vi "test_F9P_fgv-ver.vi"() -> ()   [LabVIEW 2019] (continued)
  (unwired) cluster{"X":dbl, "Y":dbl}[] [{"X"=383412.13183575624, "Y"=283542.1157386018}, {"X"=383412.14072749903, "Y"=283542.12701954495}, {"X"=383412.14072749903, "Y"=283542.12701954495}, {"X"=383412.14072749903, "Y"=283542.12701954495}, {"X"=383412.1496192395, "Y"=283542.1383004872}, {"X"=383412.1496192395, "Y"=283542.1383004872}, {"X"=383412.1496192395, "Y"=283542.1383004872}, {"X"=383412.1496192395, "Y"=283542.1383004872}, {"X"=383412.1496192395, "Y"=283542.1383004872}, {"X"=383412.1496192395, "Y"=283542.1383004872}, {"X"=383412.1589596947, "Y"=283542.1273881729}, {"X"=383412.1589596947, "Y"=283542.1273881729}, {"X"=383412.1589596947, "Y"=283542.1273881729}, {"X"=383412.1680757925, "Y"=283542.12757248693}, {"X"=383412.1683001499, "Y"=283542.11647585774}, {"X"=383412.1774162478, "Y"=283542.11666017177}, {"X"=383412.1774162478, "Y"=283542.11666017177}, {"X"=383412.1774162478, "Y"=283542.11666017177}, {"X"=383412.18675670295, "Y"=283542.10574785754}, {"X"=383412.18675670295, "Y"=283542.10574785754}, {"X"=383412.1958728009, "Y"=283542.1059321715}, {"X"=383412.1960971583, "Y"=283542.0948355424}, {"X"=383412.20521325845, "Y"=283542.09501985647}, {"X"=383412.20521325845, "Y"=283542.09501985647}, {"X"=383412.214329354, "Y"=283542.09520417044}, {"X"=383412.214329354, "Y"=283542.09520417044}, {"X"=383412.2234454518, "Y"=283542.0953884845}, {"X"=383412.2234454518, "Y"=283542.0953884845}, {"X"=383412.2234454518, "Y"=283542.0953884845}, {"X"=383412.214329354, "Y"=283542.09520417044}, {"X"=383412.214329354, "Y"=283542.09520417044}, {"X"=383412.214329354, "Y"=283542.09520417044}, {"X"=383412.2145537114, "Y"=283542.08410754264}, {"X"=383412.20543761586, "Y"=283542.08392322867}, {"X"=383412.2056619733, "Y"=283542.0728265995}, {"X"=383412.19654587307, "Y"=283542.07264228543}, {"X"=383412.19677023054, "Y"=283542.0615456572}, {"X"=383412.0980636525, "Y"=283541.9818418036}, {"X"=383411.97245749284, "Y"=283541.87939175277}, {"X"=383411.8288434909, "Y"=283541.76547644875}, {"X"=383411.64966251695, "Y"=283541.6064373785}, {"X"=383411.4077906293, "Y"=283541.390624976}, {"X"=383411.0658659977, "Y"=283541.16168851225}, {"X"=383410.6785852051, "Y"=283540.920733869}, {"X"=383410.30953659787, "Y"=283540.6801478684}, {"X"=383409.922704477, "Y"=283540.41700000333}, {"X"=383409.49985664326, "Y"=283540.1309216538}, {"X"=383409.04943613, "Y"=283539.85538702144}, {"X"=383408.5990155877, "Y"=283539.5798524129}, {"X"=383408.15771112393, "Y"=283539.30450213735}, {"X"=383407.7252983808, "Y"=283539.0404328218}, {"X"=383407.30200171185, "Y"=283538.7765478377}, {"X"=383406.8962641739, "Y"=283538.54632137535}, {"X"=383406.4998670677, "Y"=283538.3051826139}, {"X"=383406.10369428596, "Y"=283538.05294724106}, {"X"=383405.6895136327, "Y"=283537.7892466443}, {"X"=383405.28444905346, "Y"=283537.52573037276}, {"X"=383404.870044003, "Y"=283537.2731264438}, {"X"=383404.4554145847, "Y"=283537.0316191623}, {"X"=383404.04100949224, "Y"=283536.77901527355}, {"X"=383403.6266043726, "Y"=283536.52641140413}, {"X"=383403.18529961235, "Y"=283536.2510613829}, {"X"=383402.7346543793, "Y"=283535.9866237099}, {"X"=383402.29312522465, "Y"=283535.72237036366}, {"X"=383401.85182039154, "Y"=283535.44702041155}, {"X"=383401.43763949943, "Y"=283535.18332001864}, {"X"=383401.0603716887, "Y"=283534.89816360164}, {"X"=383400.74758961983, "Y"=283534.58100742893}, {"X"=383400.4815097676, "Y"=283534.2092896391}, {"X"=383400.280140006, "Y"=283533.79447545746}, {"X"=383400.14348033105, "Y"=283533.33656487794}, {"X"=383400.07197944535, "Y"=283532.81336464395}, {"X"=383400.0834208813, "Y"=283532.24743661174}, {"X"=383400.18602339644, "Y"=283531.68335159513}, {"X"=383400.41512973054, "Y"=283531.17732994177}, {"X"=383400.72426198516, "Y"=283530.7728366644}, {"X"=383401.0771800759, "Y"=283530.4580379334}, {"X"=383401.45587610855, "Y"=283530.2214685208}, {"X"=383401.88792276254, "Y"=283530.0525847101}, {"X"=383402.30928290833, "Y"=283529.9611930121}, {"X"=383402.7477535631, "Y"=283529.9256530838}, {"X"=383403.16642158024, "Y"=283529.9674209622}, {"X"=383403.52904686355, "Y"=283530.07466280117}, {"X"=383403.90878262615, "Y"=283530.2377564051}, {"X"=383404.31496931607, "Y"=283530.44578945445}, {"X"=383404.7382664643, "Y"=283530.7096742769}, {"X"=383405.1704553586, "Y"=283530.9848400567}, {"X"=383405.5937524603, "Y"=283531.2487249207}, {"X"=383405.99926602206, "Y"=283531.4900479345}, {"X"=383406.3954391052, "Y"=283531.7422832877}, {"X"=383406.81828743755, "Y"=283532.02836147026}, {"X"=383407.25002750533, "Y"=283532.3257206095}, {"X"=383407.6726514358, "Y"=283532.6228954618}, {"X"=383408.0954996884, "Y"=283532.9089737058}, {"X"=383408.5456962394, "Y"=283533.19560490194}, {"X"=383408.98655230104, "Y"=283533.4931484379}, {"X"=383409.40962482896, "Y"=283533.7681301187}, {"X"=383409.81446512, "Y"=283534.0427432001}, {"X"=383410.2101892815, "Y"=283534.3171719865}, {"X"=383410.6150295247, "Y"=283534.5917851032}, {"X"=383411.02898584673, "Y"=283534.86658255244}, {"X"=383411.4431665024, "Y"=283535.1302833934}, {"X"=383411.8575714911, "Y"=283535.3828876251}, {"X"=383412.28975995193, "Y"=283535.65805376216}, {"X"=383412.7401805953, "Y"=283535.9335885495}, {"X"=383413.1632529006, "Y"=283536.20857041556}, {"X"=383413.5772090795, "Y"=283536.48336798773}, {"X"=383414.00028133026, "Y"=283536.75834989623}, {"X"=383414.47737710393, "Y"=283537.0677276065}, {"X"=383414.95424848073, "Y"=283537.38820197195}, {"X"=383415.36775582953, "Y"=283537.6851928882}, {"X"=383415.72634217737, "Y"=283537.9921745477}, {"X"=383416.0202183364, "Y"=283538.3422525123}, {"X"=383416.2673921541, "Y"=283538.74689204094}, {"X"=383416.4496314275, "Y"=283539.2057244933}, {"X"=383416.54870396585, "Y"=283539.7183812282}, {"X"=383416.5472750222, "Y"=283540.24010709027}, {"X"=383416.48270647053, "Y"=283540.7272528411}, {"X"=383416.3369904831, "Y"=283541.1683532132}, {"X"=383416.1096783414, "Y"=283541.5856014671}, {"X"=383415.8103348771, "Y"=283541.95698867145}, {"X"=383415.43006836623, "Y"=283542.2712338854}, {"X"=383414.9873353622, "Y"=283542.51760912524}, {"X"=383414.50993287616, "Y"=283542.67447409057}, {"X"=383414.0436657404, "Y"=283542.73165373795}, {"X"=383413.5880852258, "Y"=283542.7113413258}, {"X"=383413.1160673846, "Y"=283542.60188727773}, {"X"=383412.6638522345, "Y"=283542.41512548324}, {"X"=383412.2316641198, "Y"=283542.1399593133}, {"X"=383412.1058336066, "Y"=283542.04860588827}, {"X"=383412.09671750874, "Y"=283542.04842157435}, {"X"=383412.1058336066, "Y"=283542.04860588827}, {"X"=383412.1149497068, "Y"=283542.04879020224}, {"X"=383412.12406580243, "Y"=283542.04897451616}, {"X"=383412.13295754296, "Y"=283542.0602554593}, {"X"=383412.13295754296, "Y"=283542.0602554593}, {"X"=383412.14207364316, "Y"=283542.06043977325}, {"X"=383412.1511897411, "Y"=283542.06062408723}, {"X"=383412.160305839, "Y"=283542.0608084012}]  # wpt_polypusan_20200714-3
  (unwired) cluster{"X":dbl, "Y":dbl}[] [{"X"=383411.932320843, "Y"=283542.5113466384}, {"X"=383411.94143694045, "Y"=283542.5115309522}, {"X"=383411.9503286807, "Y"=283542.5228118937}, {"X"=383411.95944477816, "Y"=283542.5229962075}, {"X"=383411.96856087557, "Y"=283542.5231805213}, {"X"=383411.9683365184, "Y"=283542.53427715093}, {"X"=383411.9774526181, "Y"=283542.5344614648}, {"X"=383411.9865687132, "Y"=283542.53464577853}, {"X"=383411.9956848153, "Y"=283542.5348300925}, {"X"=383411.8696299463, "Y"=283542.4545732997}, {"X"=383411.6993407283, "Y"=283542.3068151703}, {"X"=383411.54683498706, "Y"=283542.18161892693}, {"X"=383411.37654576113, "Y"=283542.0338608031}, {"X"=383411.1517842929, "Y"=283541.87390017736}, {"X"=383410.8998988804, "Y"=283541.7022899903}, {"X"=383410.62978125946, "Y"=283541.5303111862}, {"X"=383410.3509962426, "Y"=283541.33595482114}, {"X"=383410.072211214, "Y"=283541.1415984661}, {"X"=383409.7754183256, "Y"=283540.9357768668}, {"X"=383409.4697336811, "Y"=283540.71867434034}, {"X"=383409.146265533, "Y"=283540.47900994436}, {"X"=383408.83146475896, "Y"=283540.26172312885}, {"X"=383408.5526796635, "Y"=283540.0673668221}, {"X"=383408.28256195365, "Y"=283539.8953880912}, {"X"=383408.0122198793, "Y"=283539.7345059978}, {"X"=383407.7872339495, "Y"=283539.5856420879}, {"X"=383407.6249389544, "Y"=283539.4935514922}, {"X"=383407.4177365061, "Y"=283539.36724946724}, {"X"=383407.18341010157, "Y"=283539.2292978924}, {"X"=383406.9399675942, "Y"=283539.0911620164}, {"X"=383406.6513932718, "Y"=283538.92991135013}, {"X"=383406.33591933665, "Y"=283538.74591451185}, {"X"=383405.98465403315, "Y"=283538.5278905661}, {"X"=383405.6333887108, "Y"=283538.3098666383}, {"X"=383405.2641155198, "Y"=283538.080377482}, {"X"=383404.8590509454, "Y"=283537.8168612309}, {"X"=383404.4450945958, "Y"=283537.54206406383}, {"X"=383404.04025432153, "Y"=283537.2674512232}, {"X"=383403.6443057818, "Y"=283537.00411933445}, {"X"=383403.2485815608, "Y"=283536.7296908353}, {"X"=383402.85263297544, "Y"=283536.4663589834}, {"X"=383402.4389008485, "Y"=283536.18046528485}, {"X"=383402.025168696, "Y"=283535.89457160764}, {"X"=383401.6474522479, "Y"=283535.6316084193}, {"X"=383401.2877436384, "Y"=283535.38011048}, {"X"=383400.94694025436, "Y"=283535.0956912774}, {"X"=383400.62571511255, "Y"=283534.74506092304}, {"X"=383400.3509678404, "Y"=283534.35096557817}, {"X"=383400.140930653, "Y"=283533.9137738416}, {"X"=383399.99582789536, "Y"=283533.42238907877}, {"X"=383399.9518996638, "Y"=283532.8886451223}, {"X"=383399.9995811818, "Y"=283532.33455092355}, {"X"=383400.1475398879, "Y"=283531.782484042}, {"X"=383400.4042188871, "Y"=283531.26591866364}, {"X"=383400.7318076984, "Y"=283530.8506973626}, {"X"=383401.120965875, "Y"=283530.54773247044}, {"X"=383401.56325033365, "Y"=283530.32354980666}, {"X"=383402.03998015146, "Y"=283530.1999740305}, {"X"=383402.5151395754, "Y"=283530.15407467587}, {"X"=383402.9796124794, "Y"=283530.1856674368}, {"X"=383403.4247314314, "Y"=283530.2723747546}, {"X"=383403.85004773084, "Y"=283530.4363898795}, {"X"=383404.2922501598, "Y"=283530.6673534074}, {"X"=383404.74311997613, "Y"=283530.92069452035}, {"X"=383405.16664144257, "Y"=283531.17348273523}, {"X"=383405.61751120875, "Y"=283531.42682389263}, {"X"=383406.08594012377, "Y"=283531.7138235732}, {"X"=383406.5452528999, "Y"=283532.00063897157}, {"X"=383407.04013267846, "Y"=283532.33257814153}, {"X"=383407.5619120408, "Y"=283532.6872635217}, {"X"=383408.092583116, "Y"=283533.0532298735}, {"X"=383408.5968032415, "Y"=283533.37425681524}, {"X"=383409.08279111754, "Y"=283533.69491516484}, {"X"=383409.5692276718, "Y"=283533.9933802838}, {"X"=383410.10057165544, "Y"=283534.3260568743}, {"X"=383410.6854904599, "Y"=283534.7153225135}, {"X"=383411.26106875925, "Y"=283535.11550050834}, {"X"=383411.8279796103, "Y"=283535.493300969}, {"X"=383412.34998296807, "Y"=283535.83689001354}, {"X"=383412.82707883895, "Y"=283536.14626763324}, {"X"=383413.3495308398, "Y"=283536.4676634827}, {"X"=383413.89021501347, "Y"=283536.7894279925}, {"X"=383414.3762025273, "Y"=283537.11008664395}, {"X"=383414.844182165, "Y"=283537.4192800597}, {"X"=383415.32082914957, "Y"=283537.7508510744}, {"X"=383415.7781220907, "Y"=283538.1375366228}, {"X"=383416.1426834359, "Y"=283538.6000554199}, {"X"=383416.40562146157, "Y"=283539.12712650327}, {"X"=383416.53981222806, "Y"=283539.7071002825}, {"X"=383416.57305278804, "Y"=283540.31833644706}, {"X"=383416.451319649, "Y"=283540.92643920117}, {"X"=383416.2213151491, "Y"=283541.47684699734}, {"X"=383415.8748206522, "Y"=283541.92498900933}, {"X"=383415.43006836623, "Y"=283542.2712338854}, {"X"=383414.93241441366, "Y"=283542.5275998535}, {"X"=383414.4092070801, "Y"=283542.694639868}, {"X"=383413.8978081814, "Y"=283542.7287046846}, {"X"=383413.33350757346, "Y"=283542.6728906116}, {"X"=383412.79879883706, "Y"=283542.50666323025}, {"X"=383412.3112410692, "Y"=283542.2636810541}, {"X"=383412.1309383268, "Y"=283542.1601251152}, {"X"=383412.1222709437, "Y"=283542.13774754526}, {"X"=383412.1222709437, "Y"=283542.13774754526}, {"X"=383412.1316113989, "Y"=283542.12683523097}, {"X"=383412.1316113989, "Y"=283542.12683523097}, {"X"=383412.1316113989, "Y"=283542.12683523097}, {"X"=383412.1316113989, "Y"=283542.12683523097}, {"X"=383412.1316113989, "Y"=283542.12683523097}, {"X"=383412.14072749903, "Y"=283542.12701954495}, {"X"=383412.14984359685, "Y"=283542.1272038589}]  # poly pusan 20200714-2
  (unwired) cluster{"X":dbl, "Y":dbl}[] [{"X"=383409.9178374654, "Y"=283536.59810102}, {"X"=383409.927177923, "Y"=283536.58718870144}, {"X"=383409.93651838053, "Y"=283536.57627638616}, {"X"=383409.9549749438, "Y"=283536.5655483811}, {"X"=383409.96431539906, "Y"=283536.55463606486}, {"X"=383409.973655859, "Y"=283536.5437237469}, {"X"=383409.98277195997, "Y"=283536.54390805843}, {"X"=383409.9469806094, "Y"=283536.50988092675}, {"X"=383409.93831321446, "Y"=283536.4875033598}, {"X"=383409.9385375687, "Y"=283536.4764067302}, {"X"=383409.9385375687, "Y"=283536.4764067302}, {"X"=383409.93876192294, "Y"=283536.4653101011}, {"X"=383409.8578387605, "Y"=283536.40816815686}, {"X"=383409.7769156017, "Y"=283536.35102621204}, {"X"=383409.7589077463, "Y"=283536.3395609602}, {"X"=383409.73200814123, "Y"=283536.3168147713}, {"X"=383409.5792779161, "Y"=283536.20271519583}, {"X"=383409.27336874546, "Y"=283535.99670931126}, {"X"=383408.841180219, "Y"=283535.72154332086}, {"X"=383408.3816433538, "Y"=283535.4458244228}, {"X"=383408.05727756815, "Y"=283535.25054659066}, {"X"=383407.9223308085, "Y"=283535.15900892194}, {"X"=383407.94056302006, "Y"=283535.15937754087}, {"X"=383408.09396634065, "Y"=283535.2401872}, {"X"=383408.3194010837, "Y"=283535.36685785564}, {"X"=383408.61776466237, "Y"=283535.4950029968}, {"X"=383409.05421591504, "Y"=283535.55933303706}, {"X"=383409.60140653874, "Y"=283535.55929506075}, {"X"=383410.21285860625, "Y"=283535.5383540437}, {"X"=383410.69646085746, "Y"=283535.52592932346}, {"X"=383410.96971964114, "Y"=283535.5425553223}, {"X"=383411.1155773138, "Y"=283535.5455043238}, {"X"=383411.3519229675, "Y"=283535.5835863414}, {"X"=383411.5695876939, "Y"=283535.64349299634}, {"X"=383411.6963157314, "Y"=283535.69045989437}, {"X"=383411.94954744837, "Y"=283535.7954903261}, {"X"=383412.0940589766, "Y"=283535.86501911347}, {"X"=383412.17520648835, "Y"=283535.9110644512}, {"X"=383412.2472378928, "Y"=283535.95692547486}, {"X"=383412.2743618502, "Y"=283535.9685750442}, {"X"=383412.2743618502, "Y"=283535.9685750442}, {"X"=383412.2741374931, "Y"=283535.9796716734}, {"X"=383412.2741374931, "Y"=283535.9796716734}, {"X"=383412.2741374931, "Y"=283535.9796716734}, {"X"=383412.2741374931, "Y"=283535.9796716734}, {"X"=383412.2741374931, "Y"=283535.9796716734}, {"X"=383412.2741374931, "Y"=283535.9796716734}, {"X"=383412.2741374931, "Y"=283535.9796716734}, {"X"=383412.2741374931, "Y"=283535.9796716734}, {"X"=383412.2743618502, "Y"=283535.9685750442}, {"X"=383412.26524574624, "Y"=283535.9683907304}, {"X"=383412.2650213891, "Y"=283535.9794873595}, {"X"=383412.2650213891, "Y"=283535.9794873595}, {"X"=383412.2559052828, "Y"=283535.97930304566}, {"X"=383412.291920987, "Y"=283536.0022335576}, {"X"=383412.53581222554, "Y"=283536.11817631975}, {"X"=383412.77970346273, "Y"=283536.2341190897}, {"X"=383412.987578986, "Y"=283536.3271313491}, {"X"=383413.19545451214, "Y"=283536.42014361545}, {"X"=383413.367089974, "Y"=283536.5013219984}, {"X"=383413.49336927186, "Y"=283536.5704821794}, {"X"=383413.5293849731, "Y"=283536.59341269743}, {"X"=383413.5385010765, "Y"=283536.5935970126}, {"X"=383413.5567332834, "Y"=283536.5939656429}, {"X"=383413.56584938685, "Y"=283536.59414995805}, {"X"=383413.5749654926, "Y"=283536.59433427325}, {"X"=383413.71013653226, "Y"=283536.6747754009}, {"X"=383414.22324801044, "Y"=283537.0070836166}, {"X"=383414.9242078476, "Y"=283537.5208085642}, {"X"=383415.63002084335, "Y"=283538.2455538307}, {"X"=383416.1836939611, "Y"=283539.2780556692}, {"X"=383416.2779721501, "Y"=283540.4788876928}, {"X"=383415.9344532047, "Y"=283541.68196908606}, {"X"=383415.1402897733, "Y"=283542.62061217}, {"X"=383414.0938751328, "Y"=283542.95469220664}, {"X"=383413.47308307973, "Y"=283542.9865452564}, {"X"=383413.3452333581, "Y"=283542.9950614707}, {"X"=383413.3267768075, "Y"=283543.0057894686}, {"X"=383413.3174363517, "Y"=283543.01670178166}, {"X"=383413.38102467154, "Y"=283543.0290886174}, {"X"=383413.9084121501, "Y"=283543.1063586886}, {"X"=383414.70860945265, "Y"=283543.2224481709}, {"X"=383414.95384662825, "Y"=283543.2718112374}, {"X"=383414.95362226735, "Y"=283543.2829078666}, {"X"=383414.9533979065, "Y"=283543.2940044949}, {"X"=383414.9531735456, "Y"=283543.3051011227}, {"X"=383414.9169335171, "Y"=283543.29326722753}, {"X"=383414.6076593038, "Y"=283543.25371057465}, {"X"=383413.9711030325, "Y"=283543.1631320421}, {"X"=383413.3634655521, "Y"=283542.9954301012}, {"X"=383412.93972051237, "Y"=283542.7537380956}, {"X"=383412.5989177596, "Y"=283542.4693184259}, {"X"=383412.09537136485, "Y"=283542.11500134604}, {"X"=383411.53690398356, "Y"=283541.77067504416}, {"X"=383411.0869323256, "Y"=283541.47294704843}, {"X"=383410.7814720845, "Y"=283541.2447478443}, {"X"=383410.583610174, "Y"=283541.1075334294}, {"X"=383410.466222666, "Y"=283541.04965422716}, {"X"=383410.4297582683, "Y"=283541.04891697824}, {"X"=383410.41130171315, "Y"=283541.059644982}, {"X"=383410.8434899318, "Y"=283541.33481106185}, {"X"=383411.3746090679, "Y"=283541.67858437833}, {"X"=383411.8963877096, "Y"=283542.03327004256}, {"X"=383412.49042201624, "Y"=283542.42272013833}, {"X"=383413.04044630117, "Y"=283542.7335723024}, {"X"=383413.4459591501, "Y"=283542.9748956804}, {"X"=383413.81545630284, "Y"=283543.1932885606}, {"X"=383414.26654959243, "Y"=283543.4355335569}, {"X"=383414.59158803057, "Y"=283543.59752174537}, {"X"=383414.6727354587, "Y"=283543.6435671087}, {"X"=383414.6725110981, "Y"=283543.65466373705}, {"X"=383414.663395004, "Y"=283543.6544794205}, {"X"=383414.5277753554, "Y"=283543.59623153013}, {"X"=383414.39215570525, "Y"=283543.53798364184}, {"X"=383414.1751642665, "Y"=283543.4447870245}, {"X"=383413.7863131391, "Y"=283543.2815086416}, {"X"=383413.42548336374, "Y"=283543.085493336}, {"X"=383413.1546927557, "Y"=283542.94680433837}, {"X"=383412.9650495782, "Y"=283542.854160697}, {"X"=383412.7938629567, "Y"=283542.75078906}, {"X"=383412.56865281187, "Y"=283542.6130216534}, {"X"=383412.41547401866, "Y"=283542.52111528144}, {"X"=383412.37056660216, "Y"=283542.48690382455}, {"X"=383412.36167486466, "Y"=283542.47562288266}, {"X"=383412.28120048554, "Y"=283542.39628765377}, {"X"=383412.2182852302, "Y"=283542.3506109417}, {"X"=383412.2091691326, "Y"=283542.3504266277}, {"X"=383412.2093934901, "Y"=283542.33932999894}, {"X"=383412.2093934901, "Y"=283542.33932999894}, {"X"=383412.2093934901, "Y"=283542.33932999894}, {"X"=383412.2093934901, "Y"=283542.33932999894}, {"X"=383412.2463065955, "Y"=283542.3178739988}, {"X"=383412.2554226954, "Y"=283542.31805831287}, {"X"=383412.2645387931, "Y"=283542.31824262696}, {"X"=383412.2738792506, "Y"=283542.3073303115}, {"X"=383412.1665052908, "Y"=283542.2052488859}, {"X"=383411.77922457363, "Y"=283541.9642941928}, {"X"=383411.38305209693, "Y"=283541.71205857664}, {"X"=383411.10381838854, "Y"=283541.5398954449}, {"X"=383410.8697164487, "Y"=283541.3908471426}, {"X"=383410.6447306024, "Y"=283541.2419831568}, {"X"=383410.41062864766, "Y"=283541.0929348684}, {"X"=383410.14940274344, "Y"=283540.9322370196}, {"X"=383409.9155251322, "Y"=283540.77209211467}, {"X"=383409.6903149036, "Y"=283540.6343247839}, {"X"=383409.43842942733, "Y"=283540.4627146399}, {"X"=383409.24056747806, "Y"=283540.3255002548}, {"X"=383409.17765219585, "Y"=283540.27982356516}, {"X"=383409.2585753234, "Y"=283540.3369655045}, {"X"=383409.5375847504, "Y"=283540.52022520616}, {"X"=383409.8617259532, "Y"=283540.7265997316}, {"X"=383410.20365063194, "Y"=283540.95553614816}, {"X"=383410.608939274, "Y"=283541.20795602264}, {"X"=383410.995546983, "Y"=283541.4822005473}, {"X"=383411.3283555053, "Y"=283541.7109526976}, {"X"=383411.68873666425, "Y"=283541.9291611722}, {"X"=383411.95862989506, "Y"=283542.1122366382}, {"X"=383412.12070044235, "Y"=283542.2154239456}, {"X"=383412.1567161209, "Y"=283542.2383544585}, {"X"=383412.1658322186, "Y"=283542.23853877245}, {"X"=383412.1658322186, "Y"=283542.23853877245}, {"X"=383412.1749483163, "Y"=283542.2387230865}, {"X"=383412.1749483163, "Y"=283542.2387230865}, {"X"=383412.2025209692, "Y"=283542.2281793989}, {"X"=383412.2025209692, "Y"=283542.2281793989}, {"X"=383412.2025209692, "Y"=283542.2281793989}, {"X"=383412.21163706464, "Y"=283542.22836371296}, {"X"=383412.21163706464, "Y"=283542.22836371296}, {"X"=383412.22052880493, "Y"=283542.2396446566}, {"X"=383412.22052880493, "Y"=283542.2396446566}, {"X"=383412.18496184365, "Y"=283542.1945208857}, {"X"=383412.09537136485, "Y"=283542.11500134604}, {"X"=383411.9788813051, "Y"=283542.0127356099}, {"X"=383411.8530507877, "Y"=283541.9213821895}, {"X"=383411.67274803354, "Y"=283541.8178262597}, {"X"=383411.46532133967, "Y"=283541.7026207666}, {"X"=383411.29413467535, "Y"=283541.59924916073}, {"X"=383411.1767471755, "Y"=283541.54136994836}, {"X"=383411.07759187114, "Y"=283541.48385936284}, {"X"=383410.9510882701, "Y"=283541.42579584295}, {"X"=383410.80702553515, "Y"=283541.33407381136}, {"X"=383410.6173823041, "Y"=283541.24143021955}, {"X"=383410.48198695586, "Y"=283541.1720857659}, {"X"=383410.4457469139, "Y"=283541.16025188734}, {"X"=383410.43663081515, "Y"=283541.1600675751}, {"X"=383410.3557076998, "Y"=283541.1029256232}, {"X"=383410.1934127563, "Y"=283541.0108349785}, {"X"=383410.0039938697, "Y"=283540.90709477285}, {"X"=383409.7696675421, "Y"=283540.769143129}, {"X"=383409.53511685575, "Y"=283540.6422881183}, {"X"=383409.3730462501, "Y"=283540.53910085984}, {"X"=383409.2380995876, "Y"=283540.44756316737}, {"X"=383409.04912938597, "Y"=283540.3216297263}, {"X"=383408.81480303186, "Y"=283540.1836781074}, {"X"=383408.55402578035, "Y"=283540.00078705046}, {"X"=383408.26590022095, "Y"=283539.817343072}, {"X"=383407.9686585453, "Y"=283539.63371479337}, {"X"=383407.67141686263, "Y"=283539.450086526}, {"X"=383407.3743995172, "Y"=283539.2553616379}, {"X"=383407.05025820807, "Y"=283539.0489872076}, {"X"=383406.71700078365, "Y"=283538.8424284801}, {"X"=383406.3926350932, "Y"=283538.64715070394}, {"X"=383406.04159413883, "Y"=283538.41803012847}, {"X"=383405.7174527709, "Y"=283538.2116557487}, {"X"=383405.4113192408, "Y"=283538.01674662315}, {"X"=383405.0869534989, "Y"=283537.8214688956}, {"X"=383404.7810442931, "Y"=283537.615463163}, {"X"=383404.4840268283, "Y"=283537.4207383768}, {"X"=383404.21413331095, "Y"=283537.2376631467}, {"X"=383403.9440154383, "Y"=283537.06568455126}, {"X"=383403.65588969685, "Y"=283536.8822407282}, {"X"=383403.36753959535, "Y"=283536.70989354217}, {"X"=383403.0525142093, "Y"=283536.5037035683}, {"X"=383402.692581331, "Y"=283536.26330219803}, {"X"=383402.3237566754, "Y"=283536.0116199123}, {"X"=383401.990947726, "Y"=283535.7828681109}, {"X"=383401.75729418325, "Y"=283535.61162680085}, {"X"=383401.6312391361, "Y"=283535.5313701584}, {"X"=383401.4962923195, "Y"=283535.4398325877}, {"X"=383401.2984301499, "Y"=283535.30261838617}, {"X"=383401.0827844499, "Y"=283535.1428423272}, {"X"=383400.8944870562, "Y"=283534.98361918115}, {"X"=383400.70641399856, "Y"=283534.8132994113}, {"X"=383400.5010060944, "Y"=283534.5982245295}, {"X"=383400.3060603416, "Y"=283534.3167541855}, {"X"=383400.13958460063, "Y"=283533.9803536106}, {"X"=383400.00157887576, "Y"=283533.5890228039}, {"X"=383399.91049971955, "Y"=283533.1320337348}, {"X"=383399.89302243193, "Y"=283532.64322919585}, {"X"=383399.93890921294, "Y"=283532.17790802126}, {"X"=383400.04703835654, "Y"=283531.79155335313}, {"X"=383400.18049675727, "Y"=283531.50562124373}, {"X"=383400.30304432334, "Y"=283531.3082778588}, {"X"=383400.38800574763, "Y"=283531.1656804091}, {"X"=383400.50053984235, "Y"=283531.0125392357}, {"X"=383400.68712452496, "Y"=283530.8053893417}, {"X"=383400.8917170911, "Y"=283530.60970468115}, {"X"=383401.1596737439, "Y"=283530.43750339915}, {"X"=383401.4545300481, "Y"=283530.2880482896}, {"X"=383401.78517776896, "Y"=283530.17262028495}, {"X"=383402.16984912794, "Y"=283530.09158799663}, {"X"=383402.58052275726, "Y"=283530.07768840576}, {"X"=383402.9811828962, "Y"=283530.1079910402}, {"X"=383403.37115650147, "Y"=283530.2157857858}, {"X"=383403.8138076402, "Y"=283530.42455603235}, {"X"=383404.3193741375, "Y"=283530.6790029523}, {"X"=383404.7793600638, "Y"=283530.93252837134}, {"X"=383405.14863357117, "Y"=283531.1620174932}, {"X"=383405.4187516078, "Y"=283531.3339961164}, {"X"=383405.5988302973, "Y"=283531.4486485354}, {"X"=383405.77868462657, "Y"=283531.5743975866}, {"X"=383405.95876330684, "Y"=283531.6890500145}, {"X"=383406.19264122855, "Y"=283531.8491948027}, {"X"=383406.51633412845, "Y"=283532.0777624464}, {"X"=383406.8495918177, "Y"=283532.2843211534}, {"X"=383407.1286015494, "Y"=283532.4675807652}, {"X"=383407.4076112677, "Y"=283532.650840386}, {"X"=383407.70485319116, "Y"=283532.83446863596}, {"X"=383408.00187074905, "Y"=283533.0291935228}, {"X"=383408.3353527256, "Y"=283533.2246556581}, {"X"=383408.66838598094, "Y"=283533.44231106626}, {"X"=383408.97474396054, "Y"=283533.6261236677}, {"X"=383409.27176146646, "Y"=283533.8208486002}, {"X"=383409.61368643295, "Y"=283534.04978498194}, {"X"=383410.0009675565, "Y"=283534.2907395623}, {"X"=383410.39736476535, "Y"=283534.5318784738}, {"X"=383410.76641363365, "Y"=283534.7724644647}, {"X"=383411.117454633, "Y"=283535.0015852203}, {"X"=383411.4778360758, "Y"=283535.2197936726}, {"X"=383411.8831249549, "Y"=283535.4722135931}, {"X"=383412.2695085299, "Y"=283535.75755479146}, {"X"=383412.6385573031, "Y"=283535.9981408621}, {"X"=383412.9624742541, "Y"=283536.21561212145}, {"X"=383413.2866155505, "Y"=283536.4219867639}, {"X"=383413.62876467826, "Y"=283536.6398266781}, {"X"=383413.9800298931, "Y"=283536.85785092146}, {"X"=383414.3404111968, "Y"=283537.0760594928}, {"X"=383414.6736685308, "Y"=283537.28261850367}, {"X"=383414.979801905, "Y"=283537.47752794967}, {"X"=383415.28571090545, "Y"=283537.6835340353}, {"X"=383415.5911711697, "Y"=283537.91173338844}, {"X"=383415.88616914465, "Y"=283538.20632820437}, {"X"=383416.1620374513, "Y"=283538.5449409112}, {"X"=383416.38231168006, "Y"=283538.92683423456}, {"X"=383416.54744055454, "Y"=283539.3298149099}, {"X"=383416.64808362443, "Y"=283539.764795244}, {"X"=383416.66623305104, "Y"=283540.22030997305}, {"X"=383416.6021132184, "Y"=283540.6852624638}, {"X"=383416.4381650218, "Y"=283541.1259941986}, {"X"=383416.22930943617, "Y"=283541.53251445986}, {"X"=383415.9393064278, "Y"=283541.89298934815}, {"X"=383415.58638820087, "Y"=283542.2077875092}, {"X"=383415.21680833364, "Y"=283542.4445406474}, {"X"=383414.83945855283, "Y"=283542.6145297139}, {"X"=383414.4547875691, "Y"=283542.6955614495}, {"X"=383414.0258822629, "Y"=283542.70909185003}, {"X"=383413.5434021757, "Y"=283542.6660332347}, {"X"=383413.0713843318, "Y"=283542.55657918955}, {"X"=383412.6456200371, "Y"=283542.41475685424}, {"X"=383412.2850145638, "Y"=283542.2076449687}, {"X"=383412.1767431755, "Y"=283542.1499500583}, {"X"=383412.1767431755, "Y"=283542.1499500583}, {"X"=383412.1767431755, "Y"=283542.1499500583}, {"X"=383412.17651881813, "Y"=283542.1610466851}, {"X"=383412.17651881813, "Y"=283542.1610466851}]  # poly pusan 20200714-1
  n1 = flat-sequence {
    tunnel: [w9] -> w1
    frame #0 {
      n2 = call "fgv_gps_config.vi"("cmd"=enum16{"read", "write"}."write", "GNSS cfg"="GNSS cfg") -> ("error out"=w9:errorcluster)  [unwired: 8 in, 1 out]
    }
  }
  n3 = call "fgv_232_F9P.vi"("cmd"=enum16{"init", "read", "write", "close"}."init", "error in"=w1) -> ("error out"=w5:errorcluster)  [unwired: 7 in, 2 out]
  n4 = while {
    shift-right: [w15] -> _
    shift-left: "" -> [w23]
    shift-right: [w22] -> _
    shift-left: cluster{"Y(E)":dbl, "X(N)":dbl}[] [] -> [w14]
    tunnel: w5 -> [w19]
    tunnel: [w20] -> w3
    stop <- "정지" stop-if-true
    n5 = call "fgv_232_F9P.vi"("cmd"=enum16{"init", "read", "write", "close"}."read", "error in"=w19) -> ("error out"=w20:errorcluster, "read_buffer"=w11:string)  [unwired: 7 in, 1 out]
    n6 = Concatenate Strings(w23, w11) -> (w17:string)
    n7 = call "sub_gnss-data_check.vi"("gnss str"=w11) -> ("GNGGA_val"=w13:bool, "TM"=w12:cluster{dbl, dbl})  [unwired: 7 in, 2 out]
    n8 = Wait (ms)(milliseconds to wait=u32 20 ("대기 시간 (ms)")) -> ()  [unwired: 1 out]
    n9 = case shown="참" w13 {
      tunnel: [w26 w29] -> w22
      tunnel: w14 -> [w26 w28]
      tunnel: w12 -> [_ w27]
      frame False {
      }
      frame True {
        n10 = Build Array (concatenate)(w28, w27) -> (w29:cluster{"Y(E)":dbl, "X(N)":dbl}[])
      }
    }
    n11 = Select(t="", s="clear", f=w17) -> (s? t:f=w15:string)
    "gps receive" <- w15
    "UTM graph" <- w14
  }
  n12 = call "fgv_232_F9P.vi"("cmd"=enum16{"init", "read", "write", "close"}."close", "error in"=w3) -> ()  [unwired: 7 in, 3 out]
